vi "TTT.vi"() -> ()   [LabVIEW 2019]
panel:
  in  "停止":bool
  out "添加的路径":path
  in  "路径":path
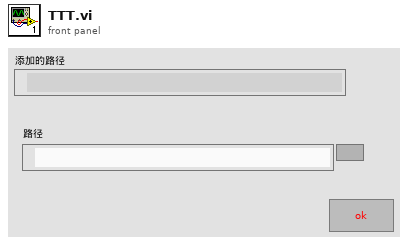
[diagram p1: front panel]
types:
  T1 = enum16{"open", "replace", "create", "open or create", "replace or create", "replace or create with confirmation"}
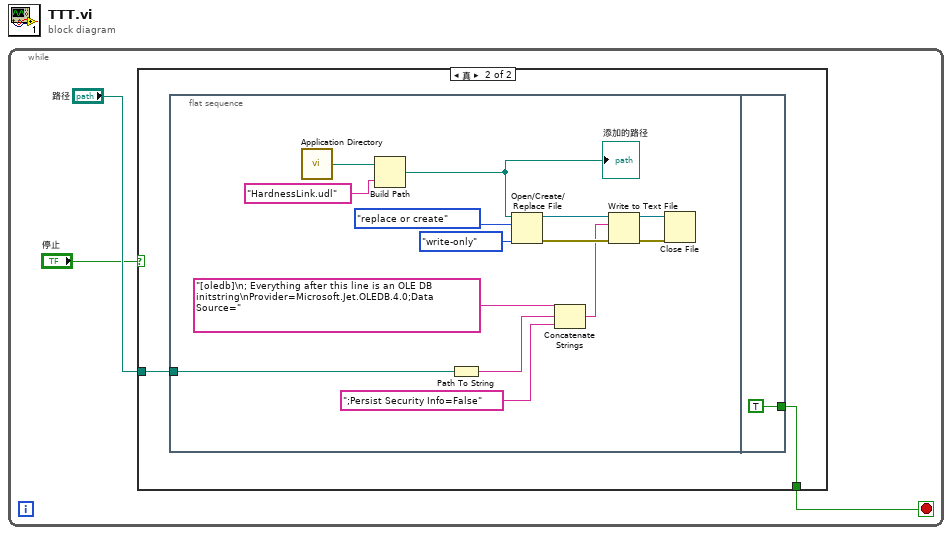
[diagram p0: block diagram]
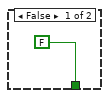
[diagram p2: hidden frame]
diagram:
  n1 = while {
    stop <- w1 stop-if-true
    n2 = case shown="真" "停止" {
      tunnel: "路径" -> [_ w6]
      tunnel: [FALSE w5] -> w1
      frame False {
      }
      frame True {
        n3 = flat-sequence {
          tunnel: w6 -> [w11]
          tunnel: [TRUE] -> w5
          frame #0 {
            n4 = call <vilib>:"Application Directory.vi"() -> ("Application Directory"=w14:path)
            n5 = Build Path(base path=w14, name or relative path="HardnessLink.udl") -> (appended path=w12:path)
            "添加的路径" <- w12
            n6 = Path To String(path=w11) -> (string=w10:string)
            n7 = Open/Create/Replace File(file path (use dialog)=w12, operation (0:open)=T1."replace or create" ("操作(0:open)"), access (0:read/write)=enum16{"read/write", "read-only", "write-only"}."write-only" ("权限(0:read/write)")) -> (refnum out=w18:refnum<file>, error out=w17:errorcluster)  [unwired: 3 in, 1 out]
            n8 = Concatenate Strings("[oledb]\n; Everything after this line is an OLE DB initstring\nProvider=Microsoft.Jet.OLEDB.4.0;Data Source=", w10, ";Persist Security Info=False" ("字符串")) -> (w8:string)
            n9 = Write to Text File(file (use dialog)=w18, text=w8, error in=w17) -> (refnum out=w15:refnum<file>, error out=w16:errorcluster)  [unwired: 1 in, 1 out]
            n10 = Close File(refnum=w15, error in=w16) -> ()  [unwired: 2 out]
          }
          frame #1 {
          }
        }
      }
    }
  }
